vi "Listbox Hide.vi"(8 "error in (no error)":errorcluster, 11 "[V] Login in":refnum<class "[V] Login.lvclass">) -> (0 "error out":errorcluster, 3 "[V] Login out":refnum<class "[V] Login.lvclass">)   [LabVIEW 2020, in "[V] Login.lvlib" / "[V] Login.lvclass"]
uses:
  [V] Login.lvclass
  [V] Login.lvclass/[V] Login.ctl
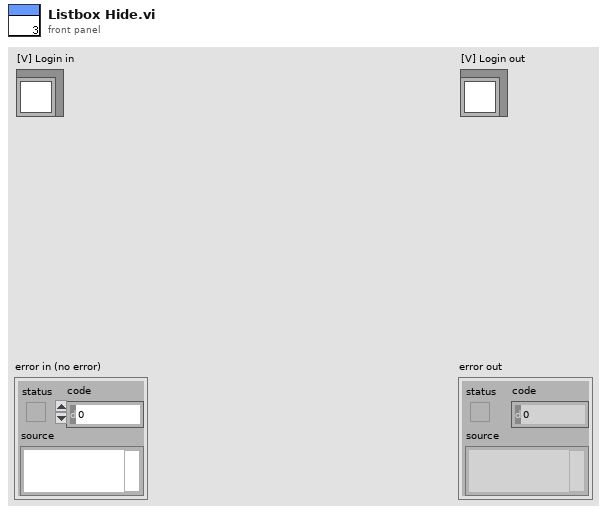
[diagram p1: front panel]
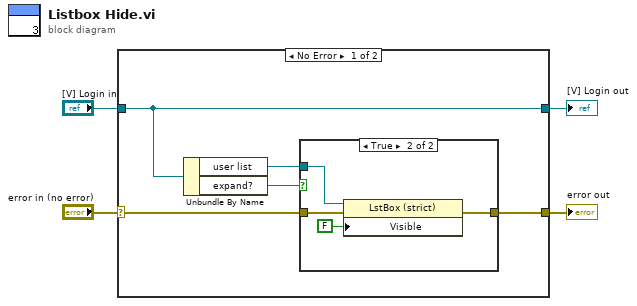
[diagram p0: block diagram]
diagram:
  n1 = case shown="No Error" "error in (no error)" {
    selector: "error in (no error)" -> [w8 w16]
    tunnel: [w6 w16] -> w3
    tunnel: [w9 w15] -> w1
    tunnel: "[V] Login in" -> [w9 w15]
    frame No Error {
      n2 = Unbundle By Name(w9) -> ("user list"=w7:refnum<vi>, "expand?"=w5:bool)
      n3 = case shown="True" w5 {
        tunnel: w8 -> [w10 w14]
        tunnel: w7 -> [_ w13]
        tunnel: [w10 w12] -> w6
        frame False {
        }
        frame True {
          n4 = property class="LstBox (strict)"(reference=w13, error in=w14, "Visible"=FALSE) -> (error out=w12:errorcluster)  [unwired: 1 out]
        }
      }
    }
    frame Error {
    }
  }
  "error out" <- w3
  "[V] Login out" <- w1
